vi "voice_learning.vi"() -> ()   [LabVIEW 2018]
uses:
  <vilib>/express/express analysis/Spectral/Block/exnSpectralBlock spectral measurements power poly.vi
  <vilib>/express/express analysis/Spectral/Block/exnSpectralBlock spectral measurements power DDT.vi
  <vilib>/express/express analysis/Spectral/XNode/ExpressSpectralMeasurementsBlockNode.xnode
panel:
  in  "Upper Cut-Off":dbl=4000.0 caption="高截止频率"
  in  "Lower Cut-Off":dbl=400.0 caption="低截止频率"
  out "Filtered Signal":dynamicdata(graph) caption="滤波后的信号"
  out "Data":dynamicdata(graph) caption="滤波前"
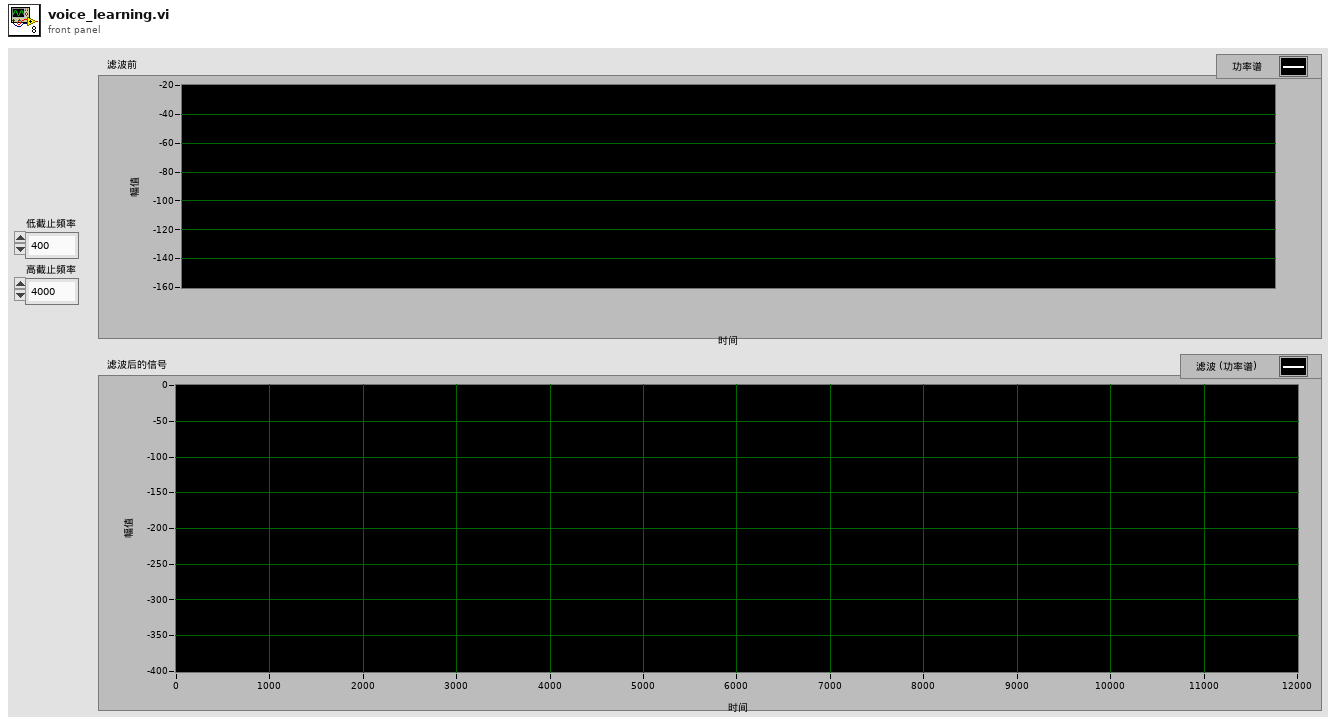
[diagram p1: front panel]
types:
  T1 = cluster{"averaging mode":u16, "weighting mode":u16, "number of averages":u32}
  T2 = cluster{"dB On (F)":bool, "unwrap phase (F)":bool, "convert to degree (F)":bool}
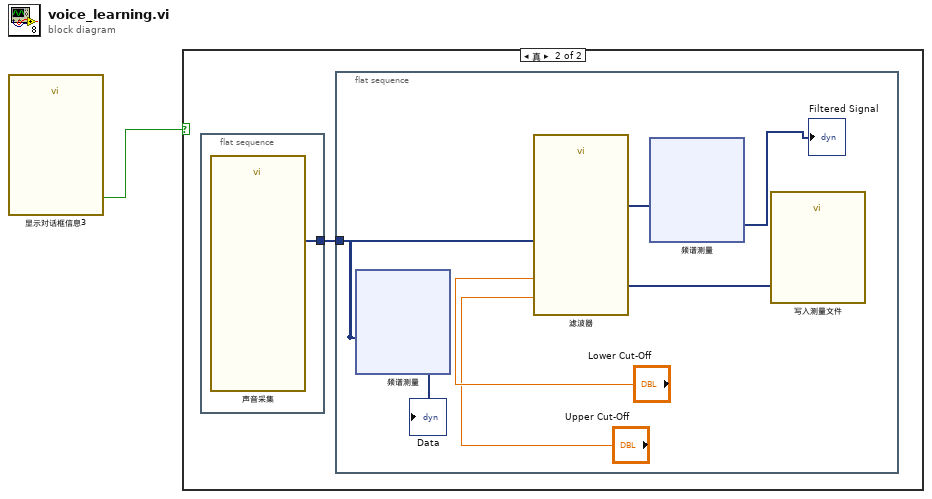
[diagram p0: block diagram]
diagram:
  n1 = call "显示对话框信息3"() -> ("确定"=w1:bool)  [unwired: 10 in, 1 out]
  n2 = case shown="真" w1 {
    frame False {
    }
    frame True {
      n3 = flat-sequence {
        tunnel: [w27] -> w2
        frame #0 {
          n4 = call "声音采集"() -> ("Data"=w27:dynamicdata)  [unwired: 18 in, 1 out]
        }
      }
      n5 = flat-sequence {
        tunnel: w2 -> [w6]
        frame #0 {
          n6 = xnode "频谱测量"("信号"=w6) -> ("功率谱"=→"Data":dynamicdata)  [unwired: 1 in, 1 out]
          n7 = call "滤波器"("Lower Cut-Off"="Lower Cut-Off", "Upper Cut-Off"="Upper Cut-Off", "Signal"=w6) -> ("Filtered Signal"=w4:dynamicdata)  [unwired: 7 in, 1 out]
          n8 = xnode "频谱测量"("信号"=w4) -> ("功率谱"=→"Filtered Signal":dynamicdata)  [unwired: 1 in, 1 out]
          n9 = call "写入测量文件"("Signals"=w4) -> ()  [unwired: 16 in, 3 out]
        }
      }
    }
  }
